vi "Reset_Encoders.vi"(8 "error in (no error)":errorcluster) -> (0 "error out":errorcluster)   [LabVIEW 2014]
uses:
  <userlib>/UCSD Robotics Lab/Robotics-Cape/LV/libroboticscape.lvlib
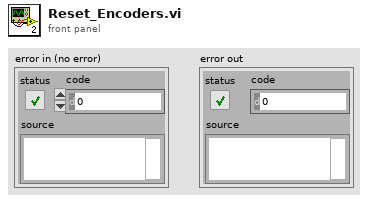
[diagram p1: front panel]
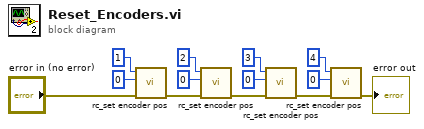
[diagram p0: block diagram]
diagram:
  n1 = call <userlib>:"rc_set encoder pos.vi"("error in (no error)"="error in (no error)", "value"=0, "ch"=1) -> ("error out"=w10:errorcluster)  [unwired: 7 in, 1 out]
  n2 = call <userlib>:"rc_set encoder pos.vi"("error in (no error)"=w10, "value"=0, "ch"=2) -> ("error out"=w11:errorcluster)  [unwired: 7 in, 1 out]
  n3 = call <userlib>:"rc_set encoder pos.vi"("error in (no error)"=w11, "value"=0, "ch"=3) -> ("error out"=w12:errorcluster)  [unwired: 7 in, 1 out]
  n4 = call <userlib>:"rc_set encoder pos.vi"("error in (no error)"=w12, "value"=0, "ch"=4) -> ("error out"=→"error out":errorcluster)  [unwired: 7 in, 1 out]
